vi "CaptStub.vi"(6 "Graph in":cluster{dbl[], dbl[]}, 7 "Index":i32, 8 "error in":errorcluster, 9 "Length":i32=250, 11 "ON":bool) -> (0 "error out":errorcluster, 2 "Values":cluster{dbl[], dbl[]})   [LabVIEW 2012]
uses:
  GlobalVariables/CalibrationState.vi
  GlobalVariables/CalibrationVolumes.vi
  GlobalVariables/Samples.vi
  GlobalVariables/AppState.vi
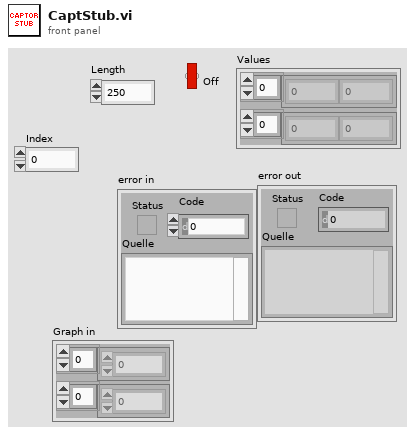
[diagram p1: front panel]
types:
  T1 = cluster{"Pressure":cluster{"TimeSamples":dbl[], "PressureSamples":dbl[]}, "Flow":cluster{"TimeSamples":dbl[], "FlowSamples":dbl[]}}
  T2 = cluster{"CalibrationVolumes":dbl[], "SetName":string}[]
  T3 = cluster{bool, "CalibrationStep":u32, "Constante":dbl[], "Gain":dbl[]}
  T4 = cluster{"CalibrationVolumes":dbl[], "SetName":string}
  T5 = cluster{"TimeSamples":dbl[], "PressureSamples":dbl[]}
  T6 = cluster{"TimeSamples":dbl[], "FlowSamples":dbl[]}
  T7 = cluster{cluster{"TimeSamples":dbl[], "PressureSamples":dbl[]}, "Flow":cluster{"TimeSamples":dbl[], "FlowSamples":dbl[]}}
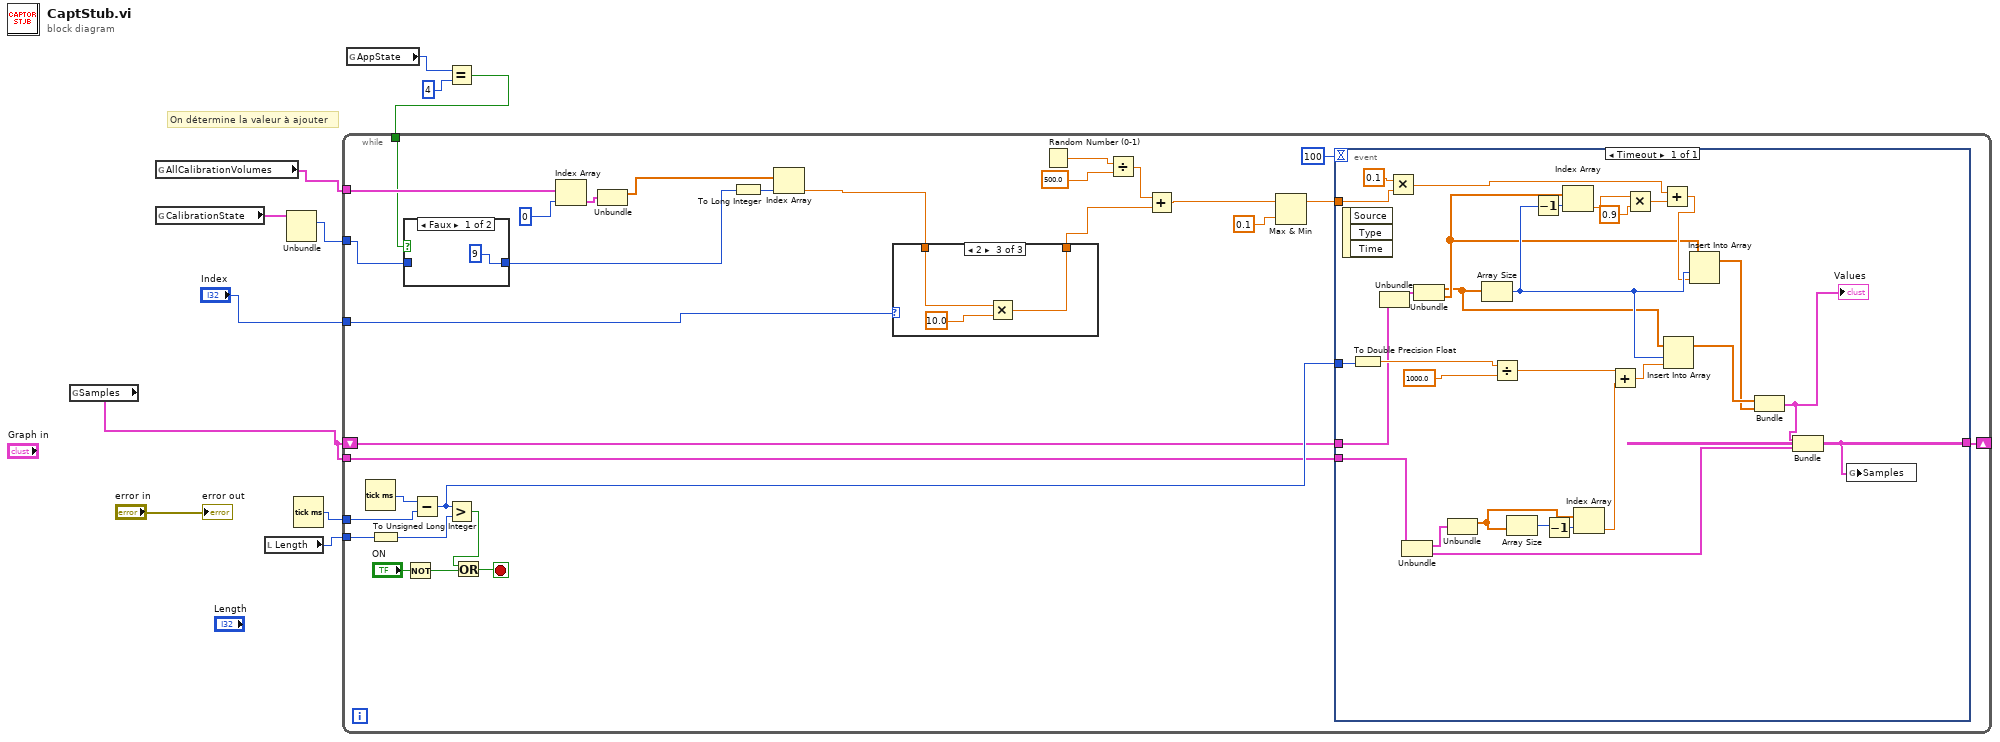
[diagram p0: block diagram]
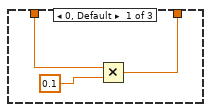
[diagram p3: hidden frame]
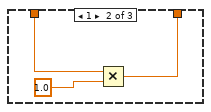
[diagram p4: hidden frame]
diagram:
  # "On détermine la valeur à ajouter"
  n1 = global read "Samples.vi" "Samples"() -> (w5:T1)
  n2 = global read "CalibrationVolumes.vi" "AllCalibrationVolumes"() -> (w7:T2)
  n3 = global read "CalibrationState.vi" "CalibrationState"() -> (w8:T3)
  n4 = local read "Length"() -> (w10:i32)
  n5 = Unbundle(w8) -> ("CalibrationStep"=w6:u32)  [unwired: 3 out]
  n6 = Tick Count (ms)() -> (millisecond timer value=w11:u32)
  n7 = global read "AppState.vi" "AppState"() -> (w2:u16)
  n8 = Equal?(x=w2, y=4) -> (x = y?=w1:bool)
  n9 = while {
    tunnel: w11 -> [w37]
    tunnel: w10 -> [w32]
    shift-right: [w30] -> _
    shift-left: w5 -> [w33]
    tunnel: w7 -> [w29]
    tunnel: w6 -> [w13]
    tunnel: w5 -> [w24]
    tunnel: "Index" -> [w18]
    tunnel: w1 -> [w15]
    stop <- w39 stop-if-true
    n10 = Tick Count (ms)() -> (millisecond timer value=w38:u32)
    n11 = To Unsigned Long Integer(number=w32) -> (unsigned 32bit integer=w31:u32)
    n12 = case shown="Faux" w15 {
      tunnel: [9 w43] -> w14
      tunnel: w13 -> [_ w43]
      frame False {
      }
      frame True {
      }
    }
    n13 = Not(x="ON") -> (.not. x?=w40:bool)
    n14 = Subtract(x=w38, y=w37) -> (x-y=w34:u32)
    n15 = Greater?(x=w34, y=w31) -> (0:w36:bool)
    n16 = Or(x=w36, y=w40) -> (x .or. y?=w39:bool)
    n17 = Index Array(array=w29, index=0) -> (element=w26:T4)
    n18 = Unbundle(w26) -> ("CalibrationVolumes"=w25:dbl[])  [unwired: 1 out]
    n19 = To Long Integer(number=w14) -> (32bit integer=w28:i32)
    n20 = Index Array(array=w25, index=w28) -> (element=w12:dbl)
    n21 = case shown="2" w18 {
      tunnel: w12 -> [w46 w47 w50]
      tunnel: [w44 w48 w51] -> w16
      frame 0, Default {
        n22 = Multiply(x=w46, y=0.1) -> (x*y=w44:dbl)
      }
      frame 1 {
        n23 = Multiply(x=w47, y=1.0) -> (x*y=w48:dbl)
      }
      frame 2 {
        n24 = Multiply(x=w50, y=10.0) -> (x*y=w51:dbl)
      }
    }
    n25 = Random Number (0-1)() -> (number: 0 to 1=w22:dbl)
    n26 = Divide(x=w22, y=500.0) -> (x/y=w21:dbl)
    n27 = Add(x=w21, y=w16) -> (x+y=w17:dbl)
    n28 = Max & Min(x=w17, y=0.1) -> (max(x,y)=w20:dbl)  [unwired: 1 out]
    n29 = event shown="[0] Timeout" {
      selector: _ -> [_]
      dyn-events: _ -> [_]
      timeout: 100 -> [_]
      tunnel: w34 -> [w76]
      tunnel: w33 -> [w73]
      tunnel: [w53] -> w30
      tunnel: w20 -> [w67]
      tunnel: w24 -> [w72]
      event Timeout {
        n30 = event-data() -> ()  [unwired: 1 in, 3 out]
        n31 = To Double Precision Float(number=w76) -> (double precision float=w75:dbl)
        n32 = Unbundle(w73) -> ("Pressure"=w57:T5)  [unwired: 1 out]
        n33 = Multiply(x=0.1, y=w67) -> (x*y=w65:dbl)
        n34 = Unbundle(w72) -> ("Pressure"=w59:T5, "Flow"=w54:T6)
        n35 = Unbundle(w57) -> ("TimeSamples"=w56:dbl[], "PressureSamples"=w58:dbl[])
        n36 = Unbundle(w59) -> ("TimeSamples"=w60:dbl[])  [unwired: 1 out]
        n37 = Array Size(array=w56) -> (size(s)=w70:i32)
        n38 = Divide(x=w75, y=1000.0) -> (x/y=w78:dbl)
        n39 = Array Size(array=w60) -> (size(s)=w81:i32)
        n40 = Decrement(x=w70) -> (x-1=w71:i32)
        n41 = Decrement(x=w81) -> (x-1=w80:i32)
        n42 = Index Array(array=w58, index=w71) -> (element=w64:dbl)
        n43 = Index Array(array=w60, index=w80) -> (element=w74:dbl)
        n44 = Add(x=w78, y=w74) -> (x+y=w77:dbl)
        n45 = Multiply(x=w64, y=0.9) -> (x*y=w66:dbl)
        n46 = Add(x=w65, y=w66) -> (x+y=w63:dbl)
        n47 = Insert Into Array(array=w56, index=w70, new element=w77) -> (w62:dbl[])
        n48 = Insert Into Array(array=w58, index=w70, new element=w63) -> (w61:dbl[])
        n49 = Bundle("TimeSamples"=w62, "PressureSamples"=w61) -> (w55:T5)  [unwired: 1 in]
        "Values" <- w55
        n50 = Bundle(w55, "Flow"=w54) -> (w53:T7)  [unwired: 1 in]
        n51 = global write "Samples.vi" "Samples"(w53) -> ()
      }
    }
  }
  "error out" <- "error in"
